vi "User.vi"() -> ()   [LabVIEW 2025]
uses:
  Cluster.ctl
  Enum.ctl
  Conn_state.ctl
  <resource>/objmgr/ni.dex.rc
panel:
  out "GSR":i32[](graph)
  out "Puls":i32[](graph)
  in  "IP":string="172.22.11.2"
  in  "Command_var":T1
  in  "stop":bool
  # "STACJA DIAGNOSTYCZNA"
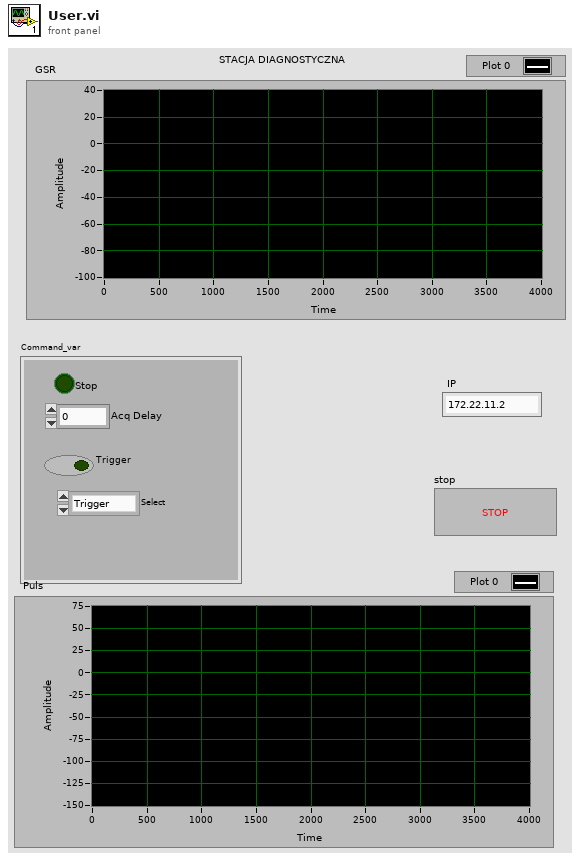
[diagram p1: front panel]
types:
  T1 = typedef "Cluster.ctl" = cluster{"Stop":bool, "Trigger":bool, "Select":T2, "Acq Delay":u16}
  T2 = typedef "Enum.ctl" = enum16{"Trigger", "Stop", "Acq_del"}
  T3 = typedef "Conn_state.ctl" = enum16{"Disconected", "Reconecting", "Connected"}
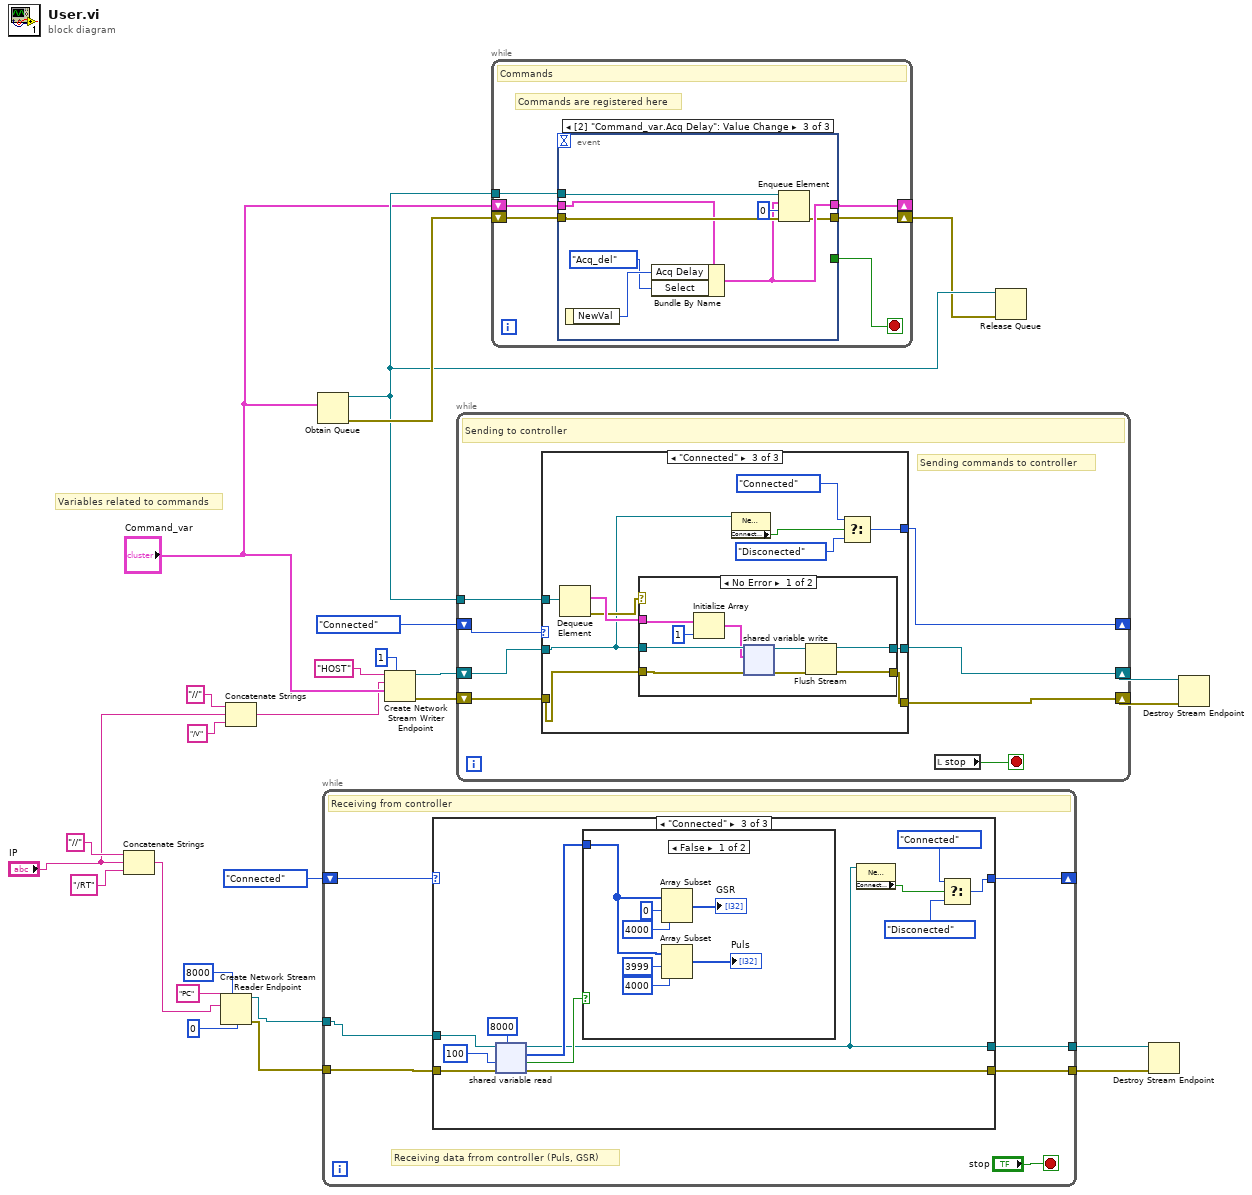
[diagram p0: block diagram]
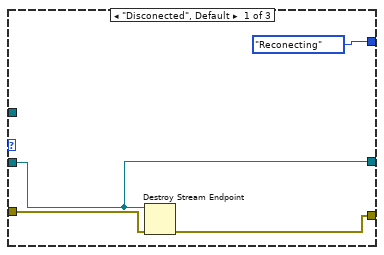
[diagram p2: hidden frame]
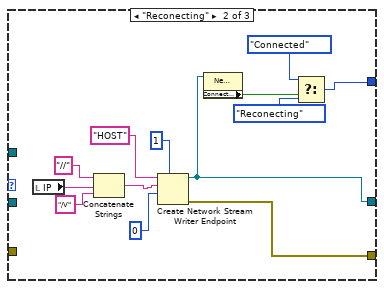
[diagram p3: hidden frame]
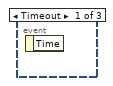
[diagram p5: hidden frame]
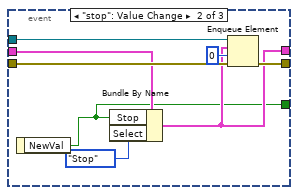
[diagram p6: hidden frame]
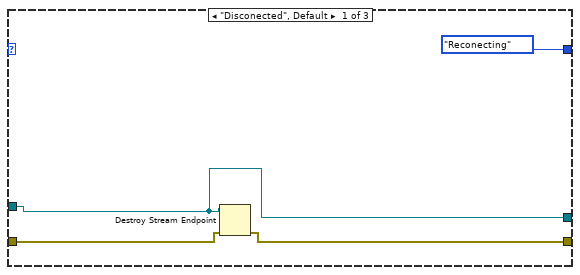
[diagram p7: hidden frame]
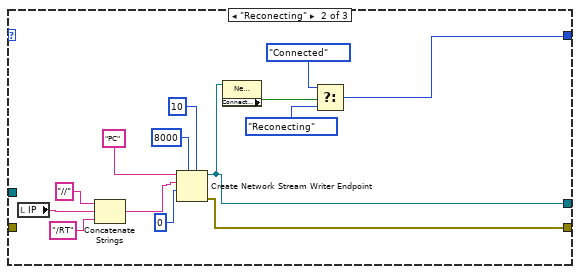
[diagram p8: hidden frame]
diagram:
  # "Variables related to commands"
  n1 = Concatenate Strings("//" ("string"), "IP", "/RT" ("string")) -> (w8:string)
  n2 = Create Network Stream Reader Endpoint(7:8000 ("reader buffer size"), 9:0, 10:w8, 11:"PC" ("reader name")) -> (0:w7:errorcluster, 3:w10:refnum<k21>)  [unwired: 3 in]
  n3 = Concatenate Strings("//" ("string"), "IP", "/V" ("string")) -> (w3:string)
  n4 = Obtain Queue(element data type="Command_var") -> (queue out=w25:refnum<queue>, error out=w26:errorcluster)  [unwired: 4 in, 1 out]
  n5 = while {
    tunnel: w10 -> [w33]
    tunnel: [w32] -> w9
    tunnel: w7 -> [w31]
    tunnel: [w30] -> w6
    shift-right: [w28] -> _
    shift-left: Conn_state."Connected" ("Conn_state") -> [w29]
    stop <- "stop" stop-if-true
    # "Receiving data frrom controller (Puls, GSR)"
    # "Receiving from controller"
    n6 = case shown="\"Connected\"" w29 {
      tunnel: w33 -> [w35 _ w63]
      tunnel: [w36 w42 w62] -> w32
      tunnel: w31 -> [w37 _ w57]
      tunnel: [w35 w40 w52] -> w30
      tunnel: [Conn_state."Reconecting" ("Conn_state") w41 w53] -> w28
      frame "Disconected", Default {
        n7 = Destroy Stream Endpoint(8:w37, 11:w35) -> (0:w36:errorcluster)
      }
      frame "Reconecting" {
        n8 = local read "IP"() -> (w39:string)
        n9 = Concatenate Strings("//" ("string"), w39, "/RT" ("string")) -> (w43:string)
        n10 = Create Network Stream Writer Endpoint(5:10 ("timeout in ms (-1)"), 7:8000 ("writer buffer size"), 9:0, 10:w43, 11:"PC" ("writer name")) -> (0:w42:errorcluster, 3:w40:refnum<k21>)  [unwired: 2 in]
        n11 = property class="Network Stream Endpoint"(reference=w40) -> ("Connected"=w51:bool)  [unwired: 1 in, 2 out]
        n12 = Select(t=Conn_state."Connected" ("Conn_state"), s=w51, f=Conn_state."Reconecting" ("Conn_state")) -> (s? t:f=w41:T3)
      }
      frame "Connected" {
        n13 = shared-variable-read(w63, w57, 100 ("timeout ms (-1)"), 8000 ("# elements")) -> (w52:refnum<k21>, w62:errorcluster, w58:bool, w60:i32[])
        n14 = case shown="False" w58 {
          tunnel: w60 -> [w66 _]
          frame False {
            n15 = Array Subset(array=w66, index=0, length=4000) -> (→"GSR":i32[])
            n16 = Array Subset(array=w66, index=3999, length=4000) -> (→"Puls":i32[])
          }
          frame True {
          }
        }
        n17 = property class="Network Stream Endpoint"(reference=w52) -> ("Connected"=w56:bool)  [unwired: 1 in, 2 out]
        n18 = Select(t=Conn_state."Connected" ("Conn_state"), s=w56, f=Conn_state."Disconected" ("Conn_state")) -> (s? t:f=w53:T3)
      }
    }
  }
  n19 = Create Network Stream Writer Endpoint(7:1 ("writer buffer size"), 9:"Command_var", 10:w3, 11:"HOST" ("writer name")) -> (0:w11:errorcluster, 3:w12:refnum<k21>)  [unwired: 3 in]
  n20 = while {
    tunnel: w25 -> [w77]
    shift-right: [w75] -> w5
    shift-left: w12 -> [w76]
    shift-right: [w71] -> w24
    shift-left: w11 -> [w78]
    shift-right: [w73] -> _
    shift-left: Conn_state."Connected" ("Conn_state") -> [w74]
    stop <- w72 stop-if-true
    # "Sending commands to controller"
    # "Sending to controller"
    n21 = case shown="\"Connected\"" w74 {
      tunnel: w77 -> [_ _ w106]
      tunnel: w78 -> [w82 _ w104]
      tunnel: w76 -> [w81 _ w96]
      tunnel: [w81 w87 w103] -> w75
      tunnel: [Conn_state."Reconecting" ("Conn_state") w89 w97] -> w73
      tunnel: [w79 w88 w102] -> w71
      frame "Disconected", Default {
        n22 = Destroy Stream Endpoint(8:w82, 11:w81) -> (0:w79:errorcluster)
      }
      frame "Reconecting" {
        n23 = local read "IP"() -> (w83:string)
        n24 = Concatenate Strings("//" ("string"), w83, "/V" ("string")) -> (w84:string)
        n25 = Create Network Stream Writer Endpoint(7:1 ("writer buffer size"), 9:0, 10:w84, 11:"HOST" ("writer name")) -> (0:w88:errorcluster, 3:w87:refnum<k21>)  [unwired: 3 in]
        n26 = property class="Network Stream Endpoint"(reference=w87) -> ("Connected"=w95:bool)  [unwired: 1 in, 2 out]
        n27 = Select(t=Conn_state."Connected" ("Conn_state"), s=w95, f=Conn_state."Reconecting" ("Conn_state")) -> (s? t:f=w89:T3)
      }
      frame "Connected" {
        n28 = Dequeue Element(queue=w106) -> (element=w105:T1, error out=w101:errorcluster)  [unwired: 2 in, 2 out]
        n29 = case shown="No Error" w101 {
          tunnel: w105 -> [w115 _]
          tunnel: w104 -> [w113 _]
          tunnel: w96 -> [w112 _]
          tunnel: [w109 _] -> w103
          tunnel: [w107 _] -> w102
          frame No Error {
            n30 = Initialize Array(w115, 1 ("dimension size")) -> (w111:T1[])
            n31 = shared-variable-write(w112, w113, w111) -> (w110:refnum<k21>, w108:errorcluster)  [unwired: 1 in, 1 out]
            n32 = Flush Stream(8:w108, 11:w110) -> (0:w107:errorcluster, 3:w109:refnum<k21>)  [unwired: 2 in, 1 out]
          }
          frame Error {
          }
        }
        n33 = property class="Network Stream Endpoint"(reference=w96) -> ("Connected"=w100:bool)  [unwired: 1 in, 2 out]
        n34 = Select(t=Conn_state."Connected" ("Conn_state"), s=w100, f=Conn_state."Disconected" ("Conn_state")) -> (s? t:f=w97:T3)
      }
    }
    n35 = local read "stop"() -> (w72:bool)
  }
  n36 = while {
    tunnel: w25 -> [w121]
    shift-right: [w119] -> w23
    shift-left: w26 -> [w120]
    shift-right: [w117] -> _
    shift-left: "Command_var" -> [w118]
    stop <- w116 stop-if-true
    # "Commands are registered here"
    # "Commands"
    n37 = event shown="[2] \"Command_var.Acq Delay\": Value Change" {
      selector: _ -> [_ _ _]
      dyn-events: _ -> [_ _ _]
      timeout: _ -> [_ _ _]
      tunnel: w121 -> [_ w129 w136]
      tunnel: w120 -> [_ w127 w135]
      tunnel: [_ w128 w132] -> w119
      tunnel: w118 -> [_ w125 w134]
      tunnel: [_ w124 w133] -> w117
      tunnel: [_ w122 _] -> w116
      event Timeout {
        n38 = event-data() -> ()  [unwired: 1 in, 1 out]
      }
      event "stop": Value Change {
        n39 = event-data() -> ("NewVal"=w122:bool)  [unwired: 1 in]
        n40 = Bundle By Name(cluster=w125, "Stop"=w122, "Select"=Enum."Stop") -> (w124:T1)
        n41 = Enqueue Element(queue=w129, element=w124, timeout in ms (-1)=0, error in (no error)=w127) -> (error out=w128:errorcluster)  [unwired: 2 out]
      }
      event Value Change {
        n42 = event-data() -> ("NewVal"=w131:u16)  [unwired: 1 in]
        n43 = Bundle By Name(cluster=w134, "Acq Delay"=w131, "Select"=Enum."Acq_del") -> (w133:T1)
        n44 = Enqueue Element(queue=w136, element=w133, timeout in ms (-1)=0, error in (no error)=w135) -> (error out=w132:errorcluster)  [unwired: 2 out]
      }
    }
  }
  n45 = Release Queue(queue=w25, error in (no error)=w23) -> ()  [unwired: 1 in, 3 out]
  n46 = Destroy Stream Endpoint(8:w9, 11:w6) -> ()  [unwired: 1 out]
  n47 = Destroy Stream Endpoint(8:w24, 11:w5) -> ()  [unwired: 1 out]
